vi "updateShell.vi"(4 "error out 2":errorcluster, 5 "Result in":string) -> (0 "error out":errorcluster, 2 "Result":string)   [LabVIEW 2011]
uses:
  Variables/GlobalGetTimingsFromCamera.vi
  Utilities/globalvariables/KoherasGetSetStatus.vi
  Variables/GlobalSetGetPositionParameters.vi
  Variables/LaserParameter.vi
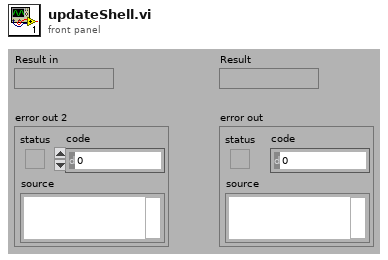
[diagram p1: front panel]
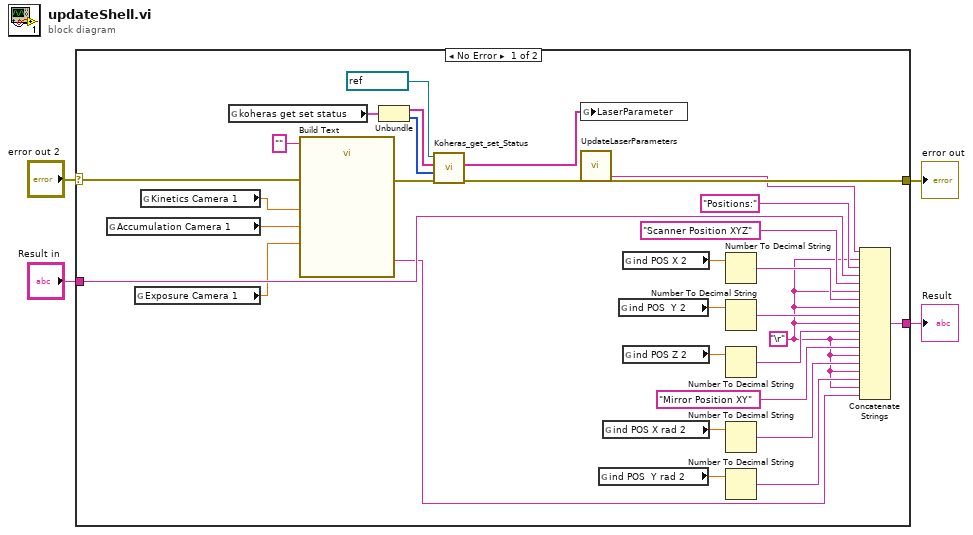
[diagram p0: block diagram]
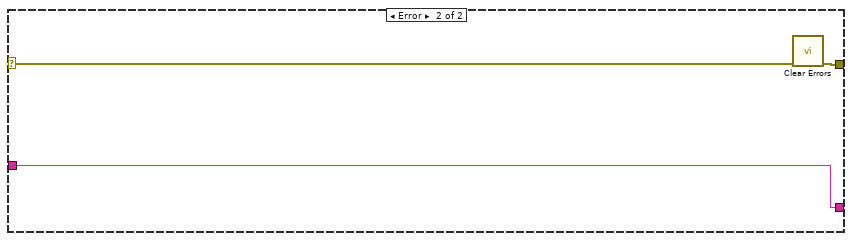
[diagram p2: hidden frame]
diagram:
  n1 = case shown="No Error" "error out 2" {
    selector: "error out 2" -> [w7 w38]
    tunnel: "Result in" -> [w35 w36]
    tunnel: [w34 w36] -> w3
    tunnel: [w21 w37] -> w1
    frame No Error {
      w12 = "\r"
      n2 = global read "GlobalGetTimingsFromCamera.vi" "Accumulation Camera 1"() -> (w11:dbl)
      n3 = global read "GlobalGetTimingsFromCamera.vi" "Exposure Camera 1"() -> (w10:dbl)
      n4 = global read "GlobalGetTimingsFromCamera.vi" "Kinetics Camera 1"() -> (w9:dbl)
      n5 = global read "KoherasGetSetStatus.vi" "koheras get set status"() -> (w17:cluster{string[], i32[]})
      n6 = call "Build Text"("Beginning Text"="", "kin"=w9, "ac"=w11, "ex"=w10, "error in (no error)"=w7) -> ("Result"=w5:string, "error out"=w6:errorcluster)  [unwired: 9 in]
      n7 = Unbundle(w17) -> (w16:string[], w15:i32[])
      n8 = call "Koheras_get_set_Status.vi"("error in"=w6, "Array 2"=w15, "Array"=w16, "VISA resource name in"=refnum<visa-resource-name> "COM3") -> ("error out"=w13:errorcluster, "Return"=w18:string[])  [unwired: 5 in, 1 out]
      n9 = global write "LaserParameter.vi" "LaserParameter"(w18) -> ()
      n10 = call "UpdateLaserParameters.vi"("error in"=w13) -> ("ToShell"=w19:string, "error out"=w21:errorcluster)  [unwired: 23 in, 2 out]
      n11 = global read "GlobalSetGetPositionParameters.vi" "ind POS  Y rad 2"() -> (w24:dbl)
      n12 = global read "GlobalSetGetPositionParameters.vi" "ind POS X rad 2"() -> (w25:dbl)
      n13 = global read "GlobalSetGetPositionParameters.vi" "ind POS  Y 2"() -> (w31:dbl)
      n14 = global read "GlobalSetGetPositionParameters.vi" "ind POS X 2"() -> (w32:dbl)
      n15 = global read "GlobalSetGetPositionParameters.vi" "ind POS Z 2"() -> (w30:dbl)
      n16 = Number To Decimal String(number=w32) -> (decimal integer string=w29:string)  [unwired: 1 in]
      n17 = Number To Decimal String(number=w31) -> (decimal integer string=w28:string)  [unwired: 1 in]
      n18 = Number To Decimal String(number=w30) -> (decimal integer string=w27:string)  [unwired: 1 in]
      n19 = Number To Decimal String(number=w25) -> (decimal integer string=w23:string)  [unwired: 1 in]
      n20 = Number To Decimal String(number=w24) -> (decimal integer string=w22:string)  [unwired: 1 in]
      n21 = Concatenate Strings(w19, w12, "Positions:" ("string"), w35, "Scanner Position XYZ" ("string"), w12, w29, w12, w28, w12, w27, w12, "Mirror Position XY" ("string"), w12, w23, w12, w22, w12, w5) -> (w34:string)
    }
    frame Error {
      n22 = call <vilib>:"Clear Errors.vi"("error in (no error)"=w38) -> ("error out"=w37:errorcluster)  [unwired: 6 in]
    }
  }
  "Result" <- w3
  "error out" <- w1
